vi "AB_RW_Project_Source_Container.vi"(7 "action":T3, 8 "error in (no error)":errorcluster, 9 "index in":i32, 10 "dataSource in":T2, 11 "buildObject":T1) -> (0 "error out":errorcluster, 1 "index out":i32, 2 "dataSource out":T2, 3 "buildObject out":T1)   [LabVIEW 2020]
doc: "Reads and writes the data to the object property bag."
uses:
  <resource>/Framework/Providers/API/ItemRef.ctl
  <vilib>/AppBuilder/RW_Project/AB_RW_Project_Source_Container_Data.ctl
  <vilib>/AppBuilder/RW_Project/AB_RW_Project_PropBag_Action.ctl
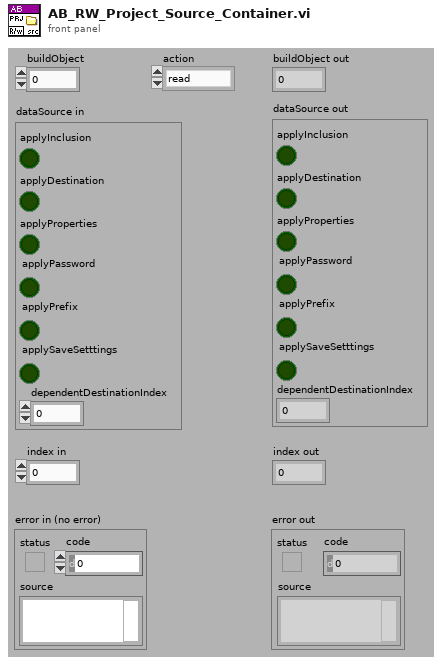
[diagram p1: front panel]
types:
  T1 = typedef "ItemRef.ctl" = u64
  T2 = typedef "AB_RW_Project_Source_Container_Data.ctl" = cluster{"applyInclusion":bool, "applyDestination":bool, "applyProperties":bool, "applyPassword":bool, "applyPrefix":bool, "applySaveSetttings":bool, "dependentDestinationIndex":i32}
  T3 = typedef "AB_RW_Project_PropBag_Action.ctl" = enum16{"read", "write", "clear", "readPrevious", "writePrevious", "clearPrevious"}
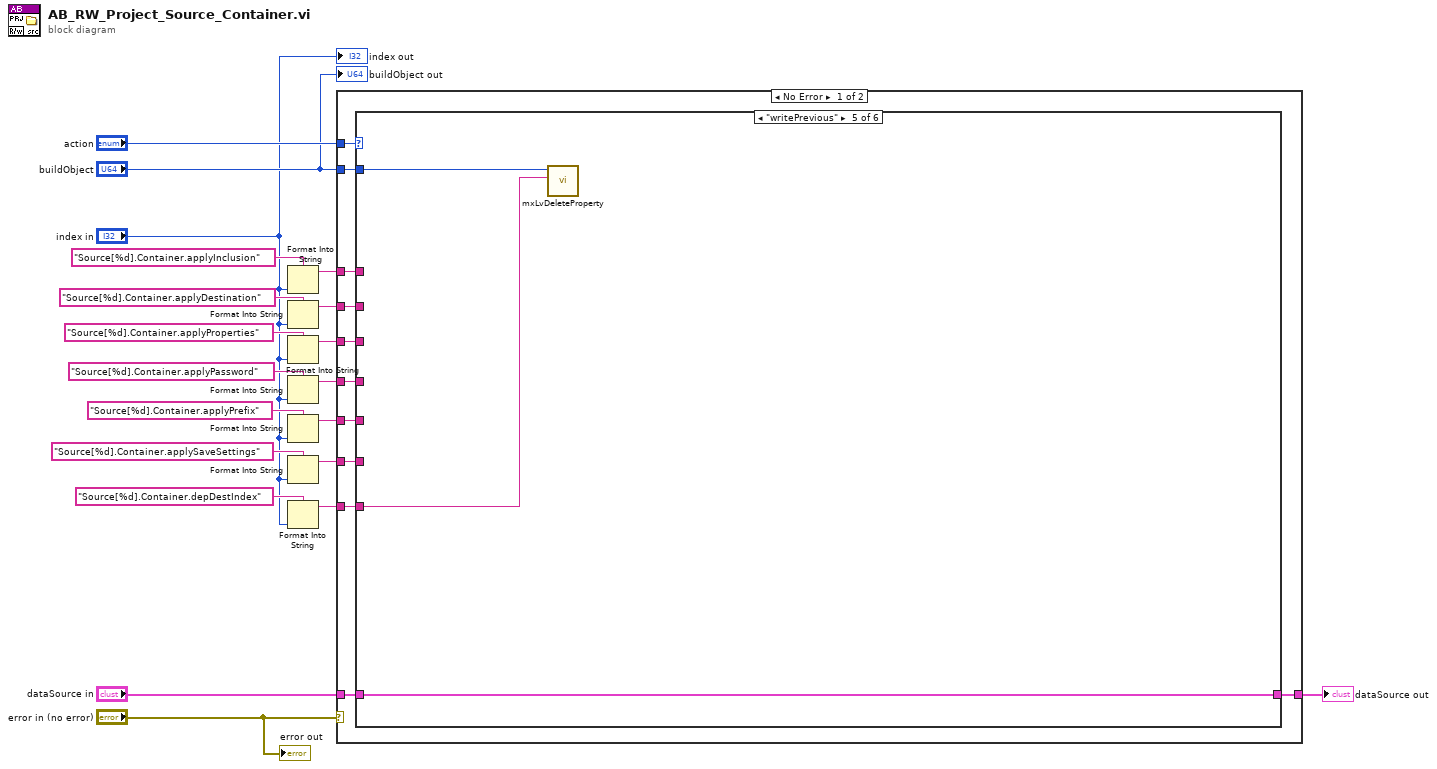
[diagram p0: block diagram]
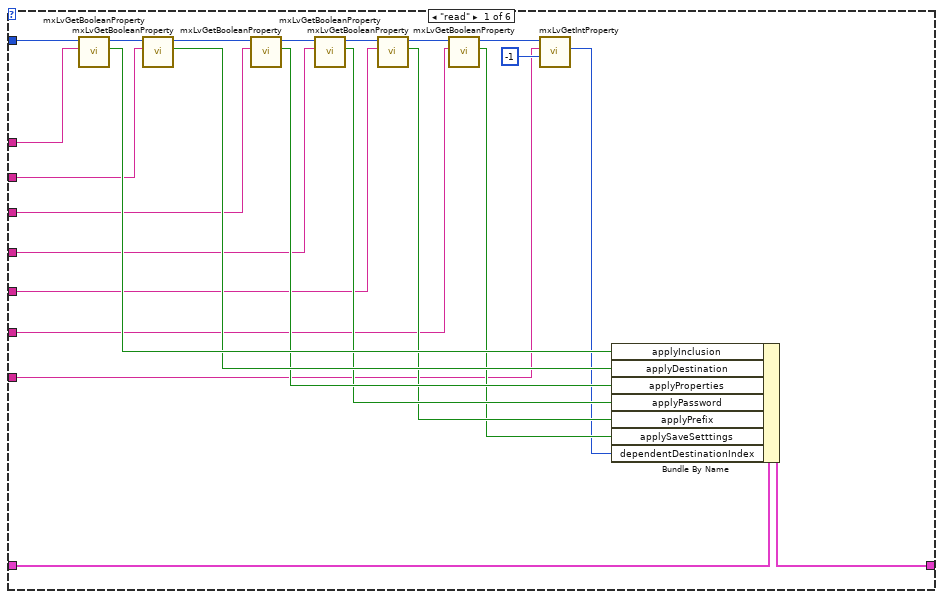
[diagram p2: hidden frame]
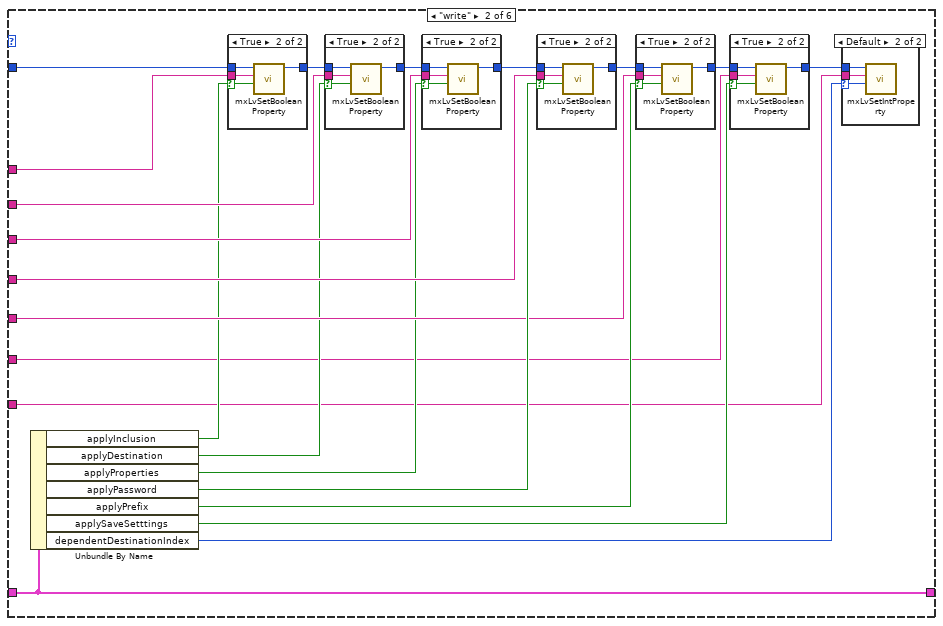
[diagram p3: hidden frame]
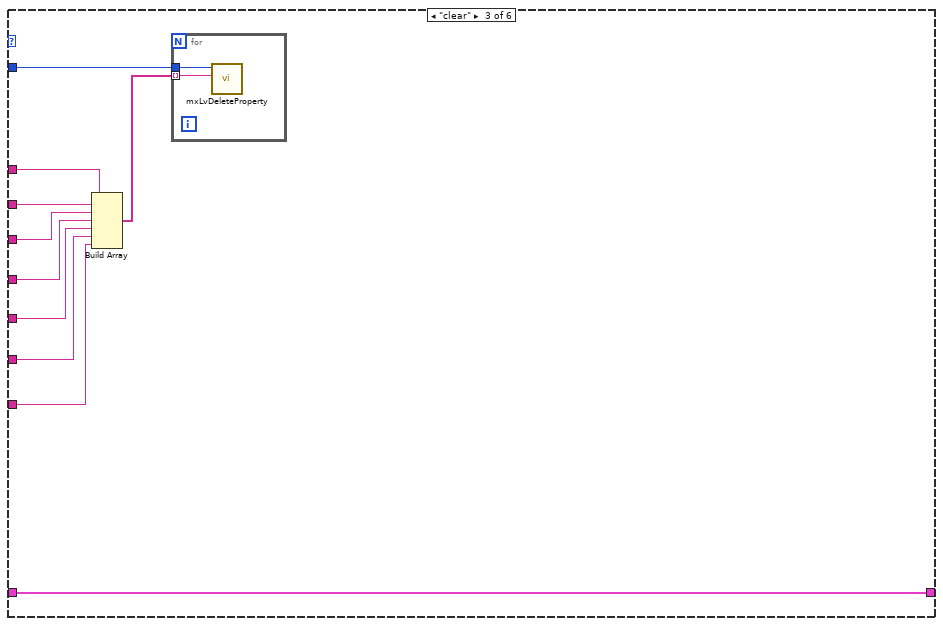
[diagram p11: hidden frame]
diagram:
  n1 = Format Into String(format string="Source[%d].Container.applyInclusion", "index in") -> (resulting string=w17:string)  [unwired: 2 in, 1 out]
  n2 = Format Into String(format string="Source[%d].Container.applyDestination", "index in") -> (resulting string=w14:string)  [unwired: 2 in, 1 out]
  n3 = Format Into String(format string="Source[%d].Container.applyProperties", "index in") -> (resulting string=w13:string)  [unwired: 2 in, 1 out]
  n4 = Format Into String(format string="Source[%d].Container.applyPassword", "index in") -> (resulting string=w8:string)  [unwired: 2 in, 1 out]
  n5 = Format Into String(format string="Source[%d].Container.applyPrefix", "index in") -> (resulting string=w6:string)  [unwired: 2 in, 1 out]
  n6 = Format Into String(format string="Source[%d].Container.applySaveSettings", "index in") -> (resulting string=w4:string)  [unwired: 2 in, 1 out]
  n7 = Format Into String(format string="Source[%d].Container.depDestIndex", "index in") -> (resulting string=w1:string)  [unwired: 2 in, 1 out]
  n8 = case shown="No Error" "error in (no error)" {
    tunnel: "action" -> [w31 _]
    tunnel: "dataSource in" -> [w30 w128]
    tunnel: w17 -> [w29 _]
    tunnel: w14 -> [w28 _]
    tunnel: w13 -> [w27 _]
    tunnel: [w26 w128] -> w12
    tunnel: "buildObject" -> [w25 _]
    tunnel: w8 -> [w24 _]
    tunnel: w6 -> [w23 _]
    tunnel: w4 -> [w22 _]
    tunnel: w1 -> [w21 _]
    frame No Error {
      n9 = case shown="\"writePrevious\"" w31 {
        tunnel: w25 -> [w53 w74 w115 _ w124 _]
        tunnel: w30 -> [w55 w77 w120 w123 w126 w127]
        tunnel: w29 -> [w51 w70 w119 _ _ _]
        tunnel: w28 -> [w48 w69 w118 _ _ _]
        tunnel: w27 -> [w46 w68 w117 _ _ _]
        tunnel: [w54 w77 w120 w123 w126 w127] -> w26
        tunnel: w24 -> [w43 w76 w114 _ _ _]
        tunnel: w23 -> [w41 w66 w113 _ _ _]
        tunnel: w22 -> [w37 w60 w112 _ _ _]
        tunnel: w21 -> [w32 w56 w111 _ w125 _]
        frame "read" {
          n10 = call <resource>:"mxLvGetBooleanProperty.vi"("Tag"=w51, "Item"=w53) -> ("Value"=w52:bool, "Item"=w50:T1)  [unwired: 7 in, 1 out]
          n11 = call <resource>:"mxLvGetBooleanProperty.vi"("Tag"=w48, "Item"=w50) -> ("Value"=w47:bool, "Item"=w49:T1)  [unwired: 7 in, 1 out]
          n12 = call <resource>:"mxLvGetBooleanProperty.vi"("Tag"=w46, "Item"=w49) -> ("Value"=w45:bool, "Item"=w44:T1)  [unwired: 7 in, 1 out]
          n13 = call <resource>:"mxLvGetBooleanProperty.vi"("Tag"=w43, "Item"=w44) -> ("Value"=w42:bool, "Item"=w40:T1)  [unwired: 7 in, 1 out]
          n14 = call <resource>:"mxLvGetBooleanProperty.vi"("Tag"=w41, "Item"=w40) -> ("Value"=w38:bool, "Item"=w39:T1)  [unwired: 7 in, 1 out]
          n15 = call <resource>:"mxLvGetBooleanProperty.vi"("Tag"=w37, "Item"=w39) -> ("Value"=w36:bool, "Item"=w34:T1)  [unwired: 7 in, 1 out]
          n16 = call <resource>:"mxLvGetIntProperty.vi"("Default Value (0)"=-1, "Tag"=w32, "Item"=w34) -> ("Value"=w33:i32)  [unwired: 6 in, 2 out]
          n17 = Bundle By Name(cluster=w55, "applyInclusion"=w52, "applyDestination"=w47, "applyProperties"=w45, "applyPassword"=w42, "applyPrefix"=w38, "applySaveSetttings"=w36, "dependentDestinationIndex"=w33) -> (w54:T2)
        }
        frame "write" {
          n18 = Unbundle By Name(w77) -> ("applyInclusion"=w65:bool, "applyDestination"=w64:bool, "applyProperties"=w63:bool, "applyPassword"=w75:bool, "applyPrefix"=w62:bool, "applySaveSetttings"=w59:bool, "dependentDestinationIndex"=w57:i32)
          n19 = case shown="True" w65 {
            selector: w65 -> [_ w103]
            tunnel: w74 -> [w101 w105]
            tunnel: w70 -> [_ w104]
            tunnel: [w101 w102] -> w73
            frame False {
            }
            frame True {
              n20 = call <resource>:"mxLvSetBooleanProperty.vi"("Value (F)"=w103, "Tag"=w104, "Item"=w105) -> ("Item"=w102:T1)  [unwired: 7 in, 1 out]
            }
          }
          n21 = case shown="True" w64 {
            selector: w64 -> [_ w98]
            tunnel: w73 -> [w96 w100]
            tunnel: w69 -> [_ w99]
            tunnel: [w96 w97] -> w67
            frame False {
            }
            frame True {
              n22 = call <resource>:"mxLvSetBooleanProperty.vi"("Value (F)"=w98, "Tag"=w99, "Item"=w100) -> ("Item"=w97:T1)  [unwired: 7 in, 1 out]
            }
          }
          n23 = case shown="True" w63 {
            selector: w63 -> [_ w93]
            tunnel: w67 -> [w91 w95]
            tunnel: w68 -> [_ w94]
            tunnel: [w91 w92] -> w72
            frame False {
            }
            frame True {
              n24 = call <resource>:"mxLvSetBooleanProperty.vi"("Value (F)"=w93, "Tag"=w94, "Item"=w95) -> ("Item"=w92:T1)  [unwired: 7 in, 1 out]
            }
          }
          n25 = case shown="True" w75 {
            selector: w75 -> [_ w108]
            tunnel: w72 -> [w106 w110]
            tunnel: w76 -> [_ w109]
            tunnel: [w106 w107] -> w71
            frame False {
            }
            frame True {
              n26 = call <resource>:"mxLvSetBooleanProperty.vi"("Value (F)"=w108, "Tag"=w109, "Item"=w110) -> ("Item"=w107:T1)  [unwired: 7 in, 1 out]
            }
          }
          n27 = case shown="True" w62 {
            selector: w62 -> [_ w88]
            tunnel: w71 -> [w86 w90]
            tunnel: w66 -> [_ w89]
            tunnel: [w86 w87] -> w61
            frame False {
            }
            frame True {
              n28 = call <resource>:"mxLvSetBooleanProperty.vi"("Value (F)"=w88, "Tag"=w89, "Item"=w90) -> ("Item"=w87:T1)  [unwired: 7 in, 1 out]
            }
          }
          n29 = case shown="True" w59 {
            selector: w59 -> [_ w83]
            tunnel: w61 -> [w81 w85]
            tunnel: w60 -> [_ w84]
            tunnel: [w81 w82] -> w58
            frame False {
            }
            frame True {
              n30 = call <resource>:"mxLvSetBooleanProperty.vi"("Value (F)"=w83, "Tag"=w84, "Item"=w85) -> ("Item"=w82:T1)  [unwired: 7 in, 1 out]
            }
          }
          n31 = case shown="Default" w57 {
            selector: w57 -> [_ w78]
            tunnel: w58 -> [_ w80]
            tunnel: w56 -> [_ w79]
            frame -1 {
            }
            frame Default {
              n32 = call <resource>:"mxLvSetIntProperty.vi"("Value (0)"=w78, "Tag"=w79, "Item"=w80) -> ()  [unwired: 7 in, 2 out]
            }
          }
        }
        frame "clear" {
          n33 = Build Array(w119, w118, w117, w114, w113, w112, w111) -> (w116:string[])
          n34 = for {
            tunnel: w115 -> [w122]
            tunnel: w116 -> [w121] mode=indexing
            n35 = call <resource>:"mxLvDeleteProperty.vi"("Tag"=w121, "Item"=w122) -> ()  [unwired: 8 in, 2 out]
          }
        }
        frame "readPrevious" {
        }
        frame "writePrevious" {
          n36 = call <resource>:"mxLvDeleteProperty.vi"("Tag"=w125, "Item"=w124) -> ()  [unwired: 8 in, 2 out]
        }
        frame "clearPrevious" {
        }
      }
    }
    frame Error {
    }
  }
  "dataSource out" <- w12
  "error out" <- "error in (no error)"
  "buildObject out" <- "buildObject"
  "index out" <- "index in"
